vi "SubPanel_RFBlock_Panel_Rev11.vi"(2 "error input":errorcluster, 3 "RF Block Input":T1) -> (0 "error output":errorcluster, 1 "RF Block Output":T1)   [LabVIEW 2019]
uses:
  Controls/RFBlockControl.ctl
panel:
  in  "RF Block Input Array":T1[](array[typedef])
  in  "VISA resource name":refnum<visa-resource-name>
  in  "Apply Configuration":bool
  in  "Frequency (GHz)":dbl
  in  "Power (dBm)":dbl
  out "Frequency (GHz) Output":dbl
  out "Power (dBm) Output":dbl
  in  "Power On?":bool
  in  "EXIT SUBVI":bool
  # "Nothing to see behind here"
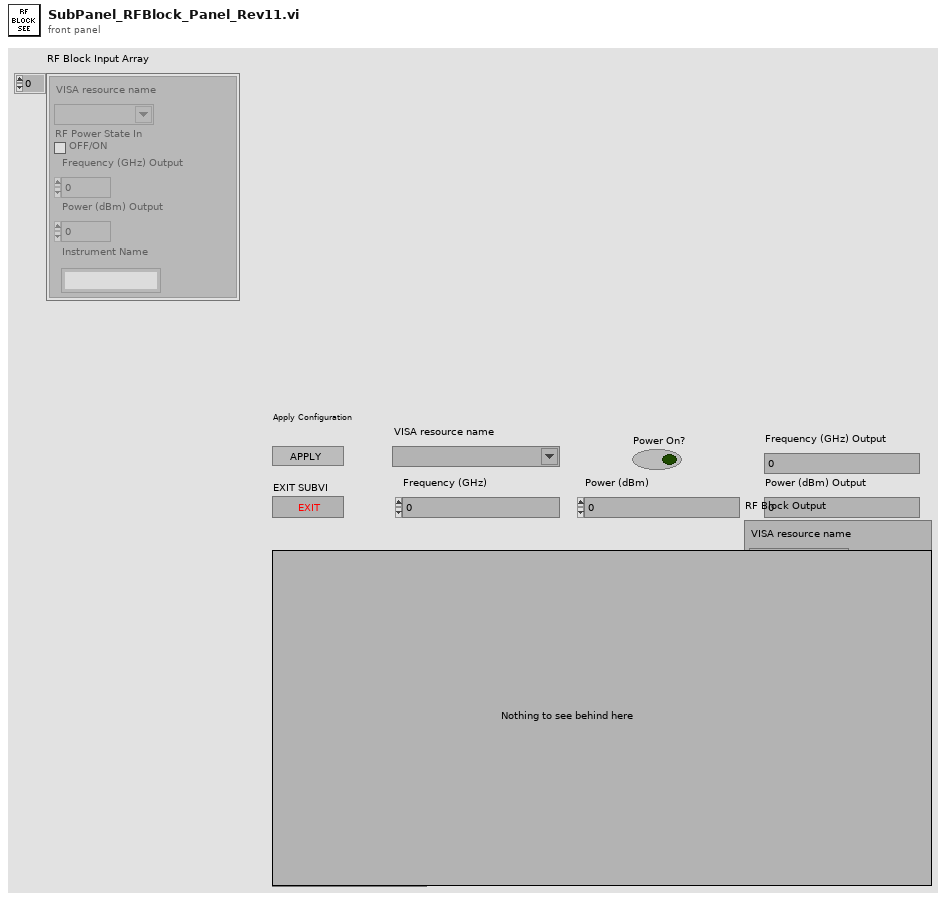
[diagram p1: front panel]
types:
  T1 = typedef "RFBlockControl.ctl" = cluster{"VISA resource name":refnum<visa-resource-name>, "RF Power State In":bool, "Frequency (GHz) Output":dbl, "Power (dBm) Output":dbl, "Instrument Name":string}
  T2 = cluster{"VISA resource name":refnum<visa-resource-name>, "Boolean out":bool, "Frequency (GHz) Output":dbl, "Power (dBm) Output":dbl}
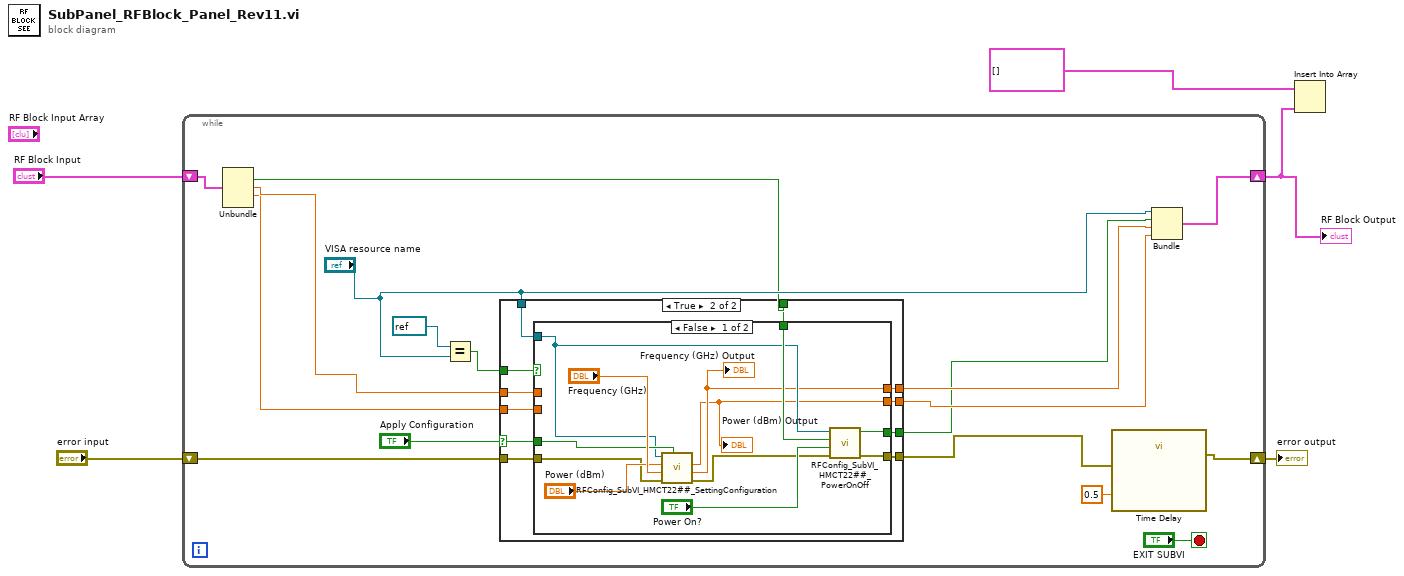
[diagram p0: block diagram]
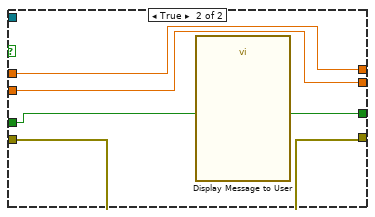
[diagram p3: hidden frame]
diagram:
  n1 = while {
    shift-right: [w9] -> w2
    shift-left: "RF Block Input" -> [w21]
    shift-right: [w11] -> w3
    shift-left: "error input" -> [w13]
    stop <- "EXIT SUBVI" stop-if-true
    n2 = Unbundle(w21) -> ("RF Power State In"=w14:bool, "Frequency (GHz) Output"=w16:dbl, "Power (dBm) Output"=w15:dbl)  [unwired: 2 out]
    n3 = Equal?(x=refnum<visa-resource-name> refnum ("VISA resource name"), y="VISA resource name") -> (x = y?=w6:bool)
    n4 = case shown="True" "Apply Configuration" {
      selector: "Apply Configuration" -> [_ w32]
      tunnel: w14 -> [w26 w37]
      tunnel: "VISA resource name" -> [_ w36]
      tunnel: [w26 w35] -> w10
      tunnel: [w25 w34] -> w12
      tunnel: w13 -> [w25 w33]
      tunnel: w6 -> [_ w31]
      tunnel: [w24 w30] -> w19
      tunnel: [w23 w29] -> w18
      tunnel: w16 -> [w24 w28]
      tunnel: w15 -> [w23 w27]
      frame False {
      }
      frame True {
        n5 = case shown="False" w31 {
          tunnel: w37 -> [w43 _]
          tunnel: w36 -> [w40 _]
          tunnel: [w45 w53] -> w35
          tunnel: [w44 w52] -> w34
          tunnel: w33 -> [w47 w52]
          tunnel: w32 -> [w46 w53]
          tunnel: [w39 w50] -> w30
          tunnel: [w38 w51] -> w29
          tunnel: w28 -> [_ w50]
          tunnel: w27 -> [_ w51]
          frame False {
            n6 = call "RFConfig_SubVI_HMCT22##_SettingConfiguration.vi"("Apply Configurations"=w46, "error in (no error)"=w47, "Frequency (GHz)"="Frequency (GHz)", "Power (dBm)"="Power (dBm)", "VISA Refnum in"=w40) -> ("error out"=w41:errorcluster, "Frequency (GHz) Output"=w39:dbl, "Power (dBm) Output"=w38:dbl)  [unwired: 4 in]
            "Frequency (GHz) Output" <- w39
            "Power (dBm) Output" <- w38
            n7 = call "RFConfig_SubVI_HMCT22##_PowerOnOff.vi"("error in (no error)"=w41, "Power On?"="Power On?", "Boolean in"=w43, "VISA Refnum in"=w40) -> ("error out"=w44:errorcluster, "Boolean out"=w45:bool)  [unwired: 6 in]
          }
          frame True {
            n8 = call "Display Message to User"() -> ()  [unwired: 10 in, 2 out]
          }
        }
      }
    }
    n9 = call "Time Delay"("error in (no error)"=w12, "Delay Time (s)"=0.5) -> ("error out"=w11:errorcluster)  [unwired: 9 in]
    n10 = Bundle("VISA resource name"="VISA resource name", "Boolean out"=w10, "Frequency (GHz) Output"=w19, "Power (dBm) Output"=w18) -> (w9:T2)  [unwired: 1 in]
  }
  "RF Block Output" <- w2
  "error output" <- w3
  n11 = Insert Into Array(array=T1[] [], new element=w2) -> ()  [unwired: 1 in, 1 out]
